vi "Write Is Change.vi"(8 "error in (no error)":errorcluster, 10 "Is Change":bool, 11 "Bundle Builder in":refnum<class "Bundle Builder.lvclass">) -> (0 "error out":errorcluster, 3 "Bundle Builder out":refnum<class "Bundle Builder.lvclass">)   [LabVIEW 2020, in "Bundle Builder.lvclass"]
uses:
  Bundle Builder.lvclass
  Bundle Builder.lvclass/Bundle Builder.ctl
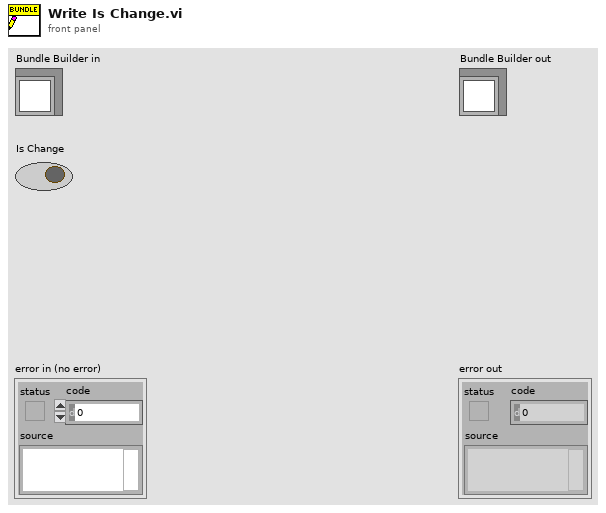
[diagram p1: front panel]
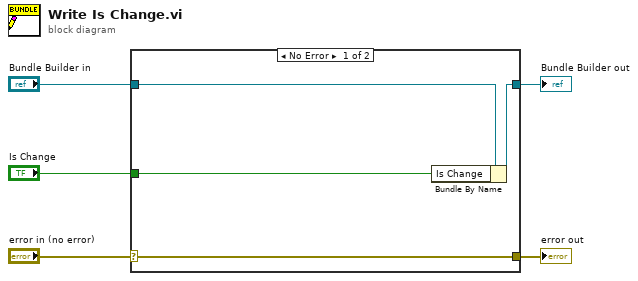
[diagram p0: block diagram]
diagram:
  n1 = case shown="No Error" "error in (no error)" {
    selector: "error in (no error)" -> [w9 w10]
    tunnel: [w9 w10] -> w4
    tunnel: [w7 w11] -> w2
    tunnel: "Bundle Builder in" -> [w8 w11]
    tunnel: "Is Change" -> [w6 _]
    frame No Error {
      n2 = Bundle By Name(cluster=w8, "Is Change"=w6) -> (w7:refnum<class "Bundle Builder.lvclass">)
    }
    frame Error {
    }
  }
  "error out" <- w4
  "Bundle Builder out" <- w2
